vi "Open Front Panel.vi"(8 "error in (no error)":errorcluster, 9 "state (Standard)":T1(ring)=enum."Standard", 10 "activate? (T)":bool=TRUE, 11 "Protected Actor Handle in":refnum<class "Protected Actor Handle.lvclass">) -> (0 "error out":errorcluster)   [LabVIEW 2020, in "AF Debug.lvlib" / "Protected Actor Handle.lvclass"]
doc: "Opens the front panel of the running actor's Actor Core clone VI."
uses:
  Protected Actor Handle.lvclass
  Protected Actor Handle.lvclass/Protected Actor Handle.ctl
  ActorFramework/Inspection API/Protected Actor Handle/Protected Actor Handle.lvclass
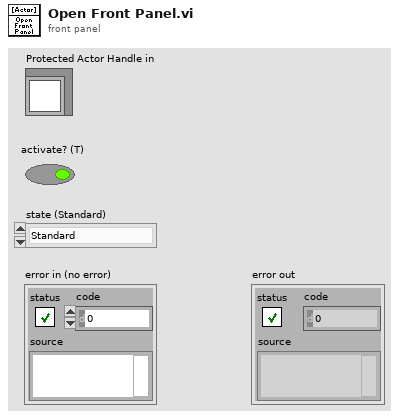
[diagram p1: front panel]
types:
  T1 = enum32{"Invalid", "Standard", "Closed", "Hidden", "Minimized", "Maximized"}
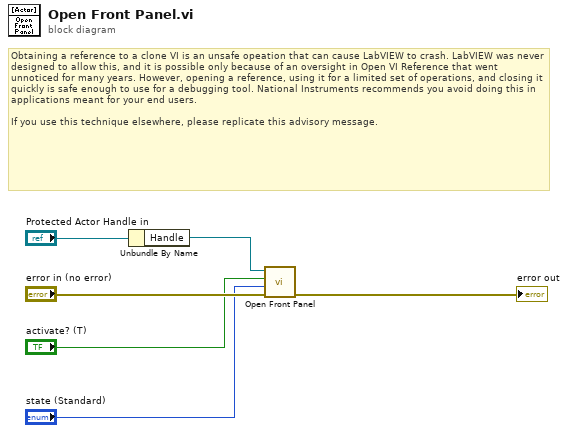
[diagram p0: block diagram]
diagram:
  # "Obtaining a reference to a clone VI is an unsafe opeation that can cause LabVIEW to crash. LabVIEW was never designed to allow this, and it is possible only because of an oversight in Open VI Reference that went unnoticed for many years. However, opening a reference, using it for a limited set of operations, and closing it quickly is safe enough to use for a debugging tool. National Instruments recommends you avoid doing this in applications meant for your end users.\n\nIf you use this technique elsewhere, please replicate this advisory message."
  n1 = Unbundle By Name("Protected Actor Handle in") -> ("Handle"=w3:refnum<class "Protected Actor Handle.lvclass">)
  n2 = call "Open Front Panel.vi"("error in (no error)"="error in (no error)", "state (Standard)"="state (Standard)", "activate? (T)"="activate? (T)", "Protected Actor Handle in"=w3) -> ("error out"=→"error out":errorcluster)  [unwired: 7 in]
